vi "Write Collision Type.vi"(10 "Edge type":T1, 11 "Ball-Edge in":refnum<class "Ball-Edge.lvclass">) -> (3 "Ball-Edge out":refnum<class "Ball-Edge.lvclass">)   [LabVIEW 2024, in "Ball-Edge.lvclass"]
doc: "MIT Licence\nCopyright (c) 2024 David Grollier"
uses:
  Ball-Edge.lvclass
  Collision type.ctl
  Ball-Edge.lvclass/Ball-Edge.ctl
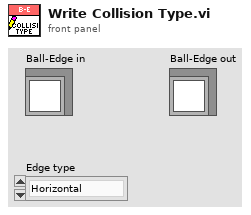
[diagram p1: front panel]
types:
  T1 = typedef "Ball-Edge.lvclass/Collision type.ctl" = enum16{"Horizontal", "Vertical", "Corner"}
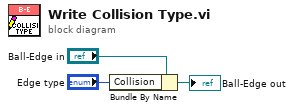
[diagram p0: block diagram]
diagram:
  n1 = Bundle By Name(cluster="Ball-Edge in", "Collision"="Edge type") -> (→"Ball-Edge out":refnum<class "Ball-Edge.lvclass">)
